vi "HEWH Gallon Target.vi"(9 "Step 2 Gallon Target":dbl, 10 "Unit Type":string(combo), 11 "Step 1A Gallon Target":dbl) -> (3 "Gallon Target":dbl)   [LabVIEW 2016]
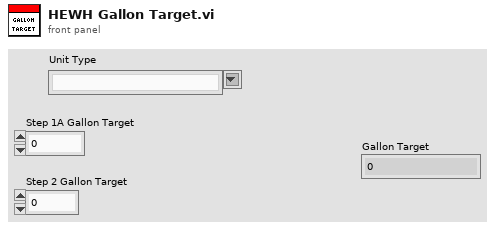
[diagram p1: front panel]
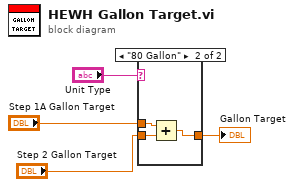
[diagram p0: block diagram]
diagram:
  n1 = case shown="\"80 Gallon\"" "Unit Type" {
    tunnel: "Step 1A Gallon Target" -> [_ w8]
    tunnel: [w5 w6] -> w2
    tunnel: "Step 2 Gallon Target" -> [w5 w7]
    frame "50 Gallon", Default {
    }
    frame "80 Gallon" {
      n2 = Add(x=w8, y=w7) -> (x+y=w6:dbl)
    }
  }
  "Gallon Target" <- w2
